vi "CanControlClose.vi"(3 "error in":errorcluster {"code" format="%.0x"}, 5 "CAN Control Handle":u32) -> (0 "error out":errorcluster {"code" format="%.0x"})   [LabVIEW 2011]
doc: "Closes the CAN controller specified by the CAN control handle."
uses:
  vcilva.dll
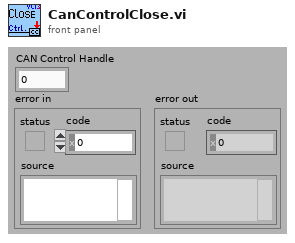
[diagram p1: front panel]
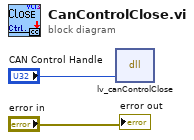
[diagram p0: block diagram]
diagram:
  n1 = dll-call lib="vcilva.dll" fn="lv_canControlClose"("hCanCtl"="CAN Control Handle") -> ()  [unwired: 5 in, 2 out]
  "error out" <- "error in"
